vi "Rename TTL.vi"(8 "error in (no error)":errorcluster, 9 "New Name":string, 10 "Old Name":string, 11 "State in":refnum<class "State.lvclass">) -> (0 "error out":errorcluster, 3 "State out":refnum<class "State.lvclass">)   [LabVIEW 2015, in "State.lvclass"]
uses:
  State.lvclass
  State.lvclass/State.ctl
  Termination/Termination.lvclass/Termination.ctl
  TTL VIs/Control Classes/Base Class/TTLController.lvclass/TTLController.ctl
  Timeout/Timeout.lvclass/Timeout.ctl
  TTL VIs/Control Classes/Base Class/Write Name.vi
  TTL VIs/Control Classes/Base Class/Read Name.vi
  Termination/Read TTL.vi
  Termination/Write TTL.vi
  Timeout/Read TTL.vi
  Timeout/Write TTL.vi
  TTL VIs/Control Classes/Base Class/TTLController.lvclass
  Timeout/Timeout.lvclass
  Termination/Termination.lvclass
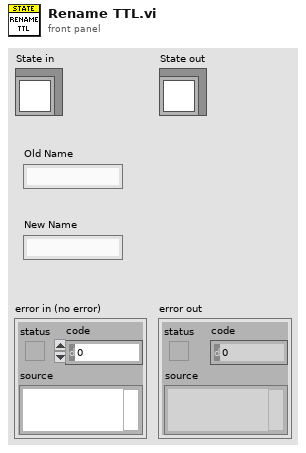
[diagram p1: front panel]
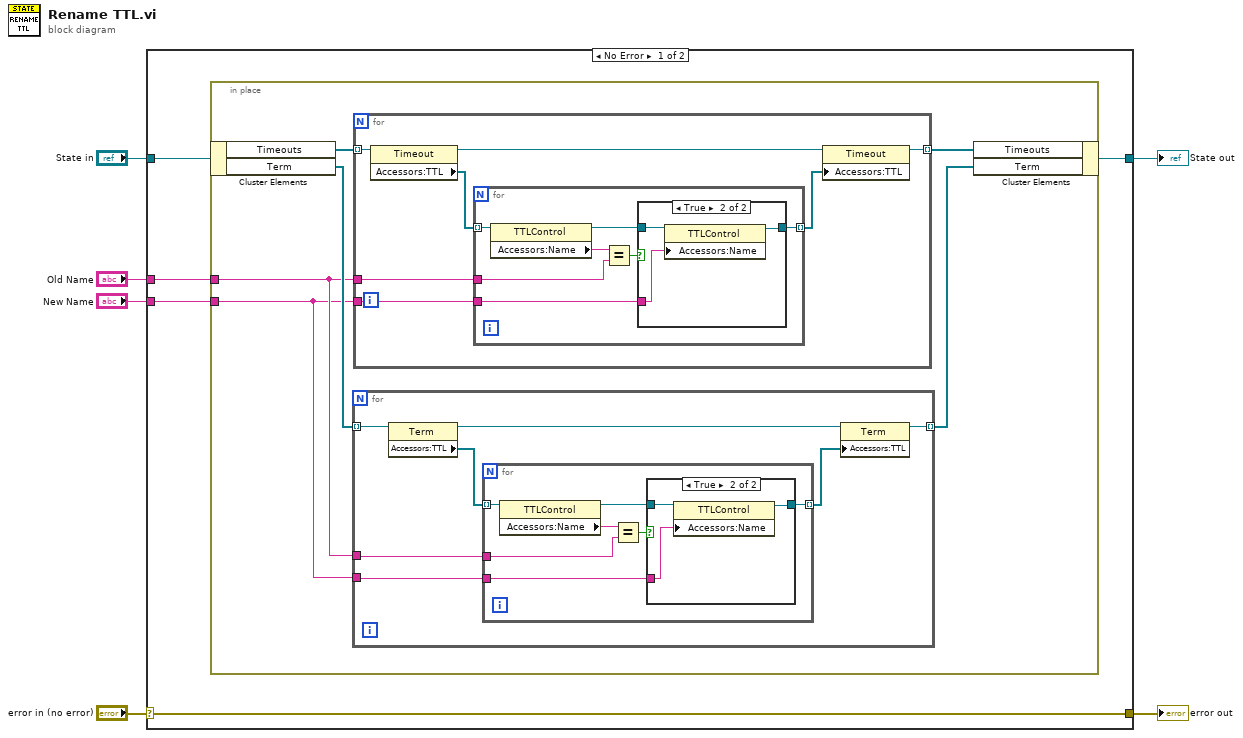
[diagram p0: block diagram]
diagram:
  n1 = case shown="No Error" "error in (no error)" {
    selector: "error in (no error)" -> [w11 w55]
    tunnel: [w11 w55] -> w5
    tunnel: [w9 w54] -> w3
    tunnel: "State in" -> [w10 w54]
    tunnel: "Old Name" -> [w8 _]
    tunnel: "New Name" -> [w7 _]
    frame No Error {
      n2 = in-place {
        in-place-border: w8 -> [w15]
        in-place-border: w7 -> [w14]
        n3 = in-place-cluster #1(w10) -> ("Timeouts"=w17:refnum<class "Timeout.lvclass">[], "Term"=w16:refnum<class "Termination.lvclass">[])
        n4 = for {
          tunnel: w16 -> [w21] mode=indexing
          tunnel: w15 -> [w19]
          tunnel: w14 -> [w18]
          tunnel: [w20] -> w12 mode=indexing
          n5 = property class="Term"(reference=w21) -> (reference out=w23:refnum<class "Termination.lvclass">, "Accessors:TTL"=w24:refnum<class "TTLController.lvclass">[])  [unwired: 1 in, 1 out]
          n6 = for {
            tunnel: w24 -> [w31] mode=indexing
            tunnel: w19 -> [w29]
            tunnel: w18 -> [w26]
            tunnel: [w25] -> w22 mode=indexing
            n7 = property class="TTLControl"(reference=w31) -> (reference out=w27:refnum<class "TTLController.lvclass">, "Accessors:Name"=w30:string)  [unwired: 1 in, 1 out]
            n8 = Equal?(x=w30, y=w29) -> (x = y?=w28:bool)
            n9 = case shown="True" w28 {
              tunnel: w27 -> [w32 w35]
              tunnel: w26 -> [_ w34]
              tunnel: [w32 w33] -> w25
              frame False {
              }
              frame True {
                n10 = property class="TTLControl"(reference=w35, "Accessors:Name"=w34) -> (reference out=w33:refnum<class "TTLController.lvclass">)  [unwired: 1 in, 1 out]
              }
            }
          }
          n11 = property class="Term"(reference=w23, "Accessors:TTL"=w22) -> (reference out=w20:refnum<class "Termination.lvclass">)  [unwired: 1 in, 1 out]
        }
        n12 = for {
          tunnel: w17 -> [w41] mode=indexing
          tunnel: w15 -> [w40]
          tunnel: w14 -> [w39]
          tunnel: [w36] -> w13 mode=indexing
          n13 = property class="Timeout"(reference=w41) -> (reference out=w38:refnum<class "Timeout.lvclass">, "Accessors:TTL"=w42:refnum<class "TTLController.lvclass">[])  [unwired: 1 in, 1 out]
          n14 = for {
            tunnel: w42 -> [w49] mode=indexing
            tunnel: w40 -> [w47]
            tunnel: w39 -> [w44]
            tunnel: [w43] -> w37 mode=indexing
            n15 = property class="TTLControl"(reference=w49) -> (reference out=w45:refnum<class "TTLController.lvclass">, "Accessors:Name"=w48:string)  [unwired: 1 in, 1 out]
            n16 = Equal?(x=w48, y=w47) -> (x = y?=w46:bool)
            n17 = case shown="True" w46 {
              tunnel: w45 -> [w50 w53]
              tunnel: w44 -> [_ w52]
              tunnel: [w50 w51] -> w43
              frame False {
              }
              frame True {
                n18 = property class="TTLControl"(reference=w53, "Accessors:Name"=w52) -> (reference out=w51:refnum<class "TTLController.lvclass">)  [unwired: 1 in, 1 out]
              }
            }
          }
          n19 = property class="Timeout"(reference=w38, "Accessors:TTL"=w37) -> (reference out=w36:refnum<class "Timeout.lvclass">)  [unwired: 1 in, 1 out]
        }
        n20 = in-place-cluster #1("Timeouts"=w13, "Term"=w12) -> (w9:refnum<class "State.lvclass">)
      }
    }
    frame Error {
    }
  }
  "error out" <- w5
  "State out" <- w3
